vi "Throw Unknown Channel Error.vi"(8 "error in (no error)":errorcluster, 10 "Missing Channel":string, 11 "Expression String in":string) -> (0 "error out":errorcluster)   [LabVIEW 2024, in "Output Sequencer.lvlib" / "Output Sequencer.lvclass"]
uses:
  Output Sequencer.lvclass
  Globals/Global Strings.vi
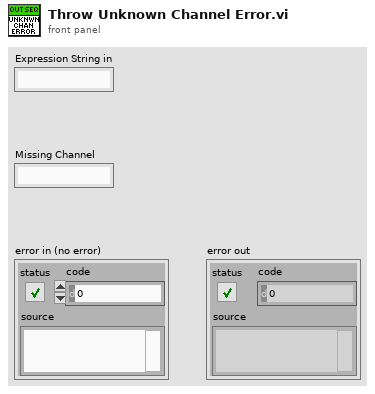
[diagram p1: front panel]
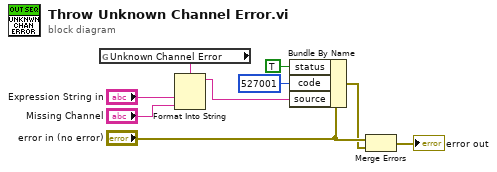
[diagram p0: block diagram]
diagram:
  n1 = global read "Global Strings.vi" "Unknown Channel Error"() -> (w9:string)
  n2 = Format Into String(format string=w9, "Expression String in", "Missing Channel") -> (resulting string=w8:string)  [unwired: 2 in, 1 out]
  n3 = Bundle By Name(cluster="error in (no error)", "status"=TRUE ("is warning? (False)"), "code"=527001 ("error code (0)"), "source"=w8) -> (w4:errorcluster)
  n4 = Merge Errors("error in (no error)", w4) -> (→"error out":errorcluster)
